vi "Joints to Angle YZ.vi"(10 "Origin Joint":cluster{"x":sgl, "y":sgl, "z":sgl}, 11 "Moving Joint":cluster{"x":sgl, "y":sgl, "z":sgl}) -> (3 "Angle":dbl)   [LabVIEW 2011]
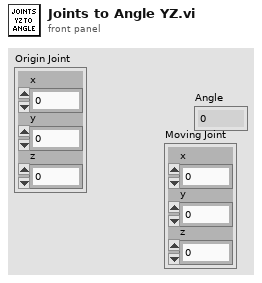
[diagram p1: front panel]
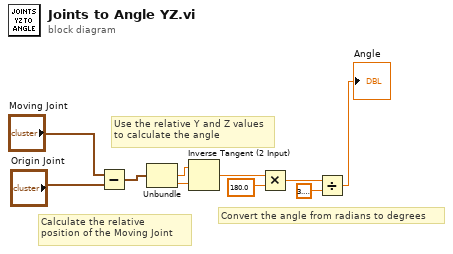
[diagram p0: block diagram]
diagram:
  # "Convert the angle from radians to degrees"
  # "Use the relative Y and Z values\nto calculate the angle"
  # "Calculate the relative\nposition of the Moving Joint"
  n1 = Subtract(x="Moving Joint", y="Origin Joint") -> (x-y=w5:cluster{"x":sgl, "y":sgl, "z":sgl})
  n2 = Unbundle(w5) -> ("y"=w3:sgl, "z"=w4:sgl)  [unwired: 1 out]
  n3 = Inverse Tangent (2 Input)(1:w4, 2:w3) -> (0:w6:sgl)
  n4 = Multiply(x=w6, y=sgl 180.0) -> (x*y=w8:sgl)
  n5 = Divide(x=w8, y=3.141592653589793) -> (x/y=→"Angle":dbl)
